vi "CSTK_BuildApplication_Manager_SaveProjectChangeLog.vi"(8 "错误输入（无错误）":errorcluster, 11 "BuildApplication Data in":T1={"Build Specification Name"="", "Destination Path"=path "", "Files Generated by Build"=[], "Exe Path Generated by Build"=path "", "Version"="", "Datatime"=timestamp(0 s since 1904-01-01), "ChangeLog"="", "Package as a ZIP file?"=TRUE, "Rename EXE File Name?"=FALSE, "Zip File Path"=path ""} {"Datatime" format="%<%.3X %x>T"}) -> (0 "错误输出":errorcluster, 3 "BuildApplication Data out":T1={"Build Specification Name"="", "Destination Path"=path "", "Files Generated by Build"=[], "Exe Path Generated by Build"=path "", "Version"="", "Datatime"=timestamp(0 s since 1904-01-01), "ChangeLog"="", "Package as a ZIP file?"=TRUE, "Rename EXE File Name?"=FALSE, "Zip File Path"=path ""} {"Datatime" format="%<%.3X %x>T"})   [LabVIEW 2015, in "CSTK_BuildApplication_Manager.lvlib"]
uses:
  CSTK_BuildApplication_Manager.lvlib
  CSTK_BuildApplication_Manager_data.ctl
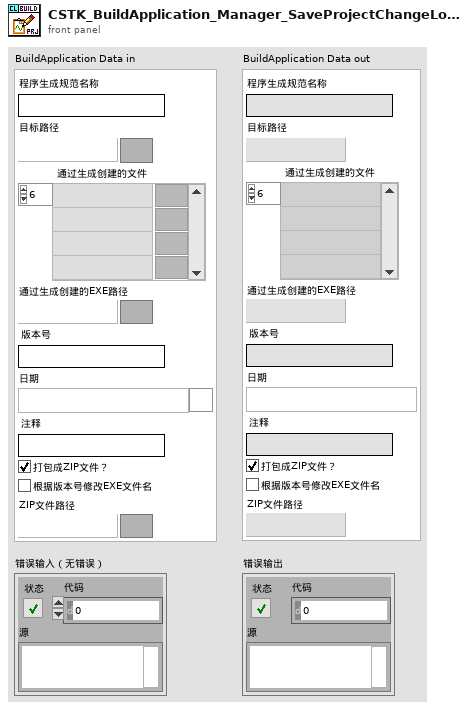
[diagram p1: front panel]
types:
  T1 = typedef "CSTK_BuildApplication_Manager.lvlib/CSTK_BuildApplication_Manager_data.ctl" = cluster{"Build Specification Name":string, "Destination Path":path, "Files Generated by Build":path[], "Exe Path Generated by Build":path, "Version":string, "Datatime":timestamp, "ChangeLog":string, "Package as a ZIP file?":bool, "Rename EXE File Name?":bool, "Zip File Path":path}
  T2 = enum16{"open", "replace", "create", "open or create", "replace or create", "replace or create with confirmation"}
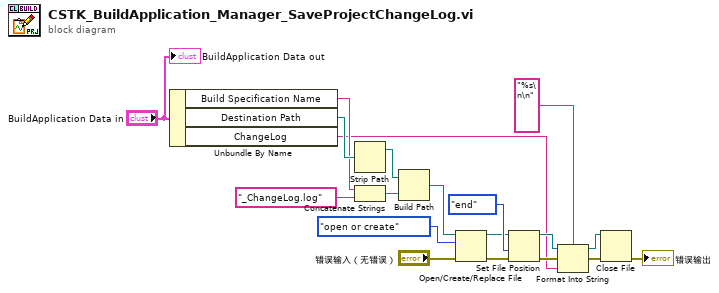
[diagram p0: block diagram]
diagram:
  n1 = Unbundle By Name("BuildApplication Data in") -> ("Build Specification Name"=w3:string, "Destination Path"=w5:path, "ChangeLog"=w2:string)
  n2 = Strip Path(path=w5) -> (stripped path=w4:path)  [unwired: 1 out]
  n3 = Concatenate Strings(w3, "_ChangeLog.log" ("字符串")) -> (w8:string)
  n4 = Build Path(base path=w4, name or relative path=w8) -> (appended path=w9:path)
  n5 = Open/Create/Replace File(file path (use dialog)=w9, error in="错误输入（无错误）", operation (0:open)=T2."open or create" ("操作(0:open)")) -> (refnum out=w11:refnum<file>, error out=w12:errorcluster)  [unwired: 3 in, 1 out]
  n6 = Set File Position(refnum=w11, from (0:start)=enum16{"start", "end", "current"}."end" ("自（0:起始）"), error in=w12) -> (refnum out=w15:refnum<file>, error out=w16:errorcluster)  [unwired: 1 in]
  n7 = Format Into String(format string="%s\n\n" ("格式字符串"), initial string=w15, error in=w16, w2) -> (resulting string=w14:refnum<file>, error out=w17:errorcluster)
  n8 = Close File(refnum=w14, error in=w17) -> (error out=→"错误输出":errorcluster)  [unwired: 1 out]
  "BuildApplication Data out" <- "BuildApplication Data in"
